vi "XB PC Close.vi"(0 "error in (no error)":errorcluster, 1 "VISA resource name":refnum<visa-resource-name>) -> ()   [LabVIEW 2014]
doc: "This VI will close the port used to communicate with a NXT using XBee."
uses:
  <vilib>/Instr/_visa.llb/VISA Flush IO Buffer Mask.ctl
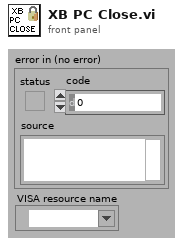
[diagram p1: front panel]
types:
  T1 = typedef "VISA Flush IO Buffer Mask.ctl" = u16
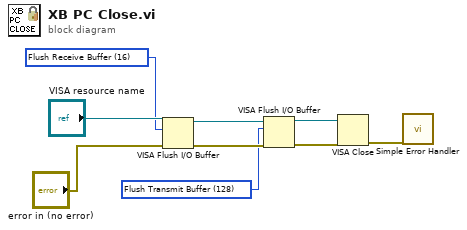
[diagram p0: block diagram]
diagram:
  w1 = T1 128 items=["Flush Receive Buffer"=16, "Write Transmit Buffer to Device"=32, "Flush Receive Buffer (No I/O)"=64, "Flush Transmit Buffer"=128] ("Mask")
  w2 = T1 16 items=["Flush Receive Buffer"=16, "Write Transmit Buffer to Device"=32, "Flush Receive Buffer (No I/O)"=64, "Flush Transmit Buffer"=128] ("Mask")
  n1 = VISA Flush I/O Buffer(VISA resource name="VISA resource name", mask (16)=w2, error in (no error)="error in (no error)") -> (VISA resource name out=w7:refnum<visa-resource-name>, error out=w4:errorcluster)
  n2 = VISA Flush I/O Buffer(VISA resource name=w7, mask (16)=w1, error in (no error)=w4) -> (VISA resource name out=w6:refnum<visa-resource-name>, error out=w3:errorcluster)
  n3 = VISA Close(VISA resource name=w6, error in (no error)=w3) -> (error out=w9:errorcluster)
  n4 = call <vilib>:"Simple Error Handler.vi"("error in (no error)"=w9) -> ()  [unwired: 1 in, 8 out]
